vi "Tosca-Initialize Digital Inputs.vi"(7 "Action":enum16{"Stop", "Preview", "Run"}(ring), 11 "error in (no error)":errorcluster) -> (4 "Digital Inputs out":T1[](array[typedef]), 15 "error out":errorcluster)   [LabVIEW 2020]
uses:
  Tosca-Digital Input.ctl
  Sub VIs/Tosca-Globals.vi
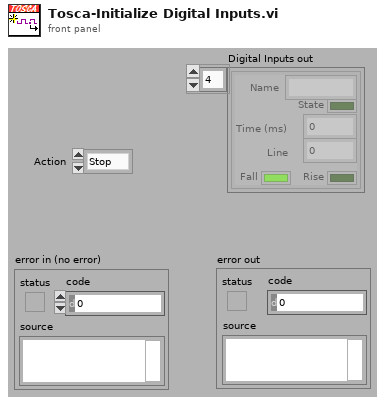
[diagram p1: front panel]
types:
  T1 = typedef "Tosca-Digital Input.ctl" = cluster{"Name":string, "State":bool, "Time (ms)":dbl, "Line":i32, "Rise":bool, "Fall":bool}
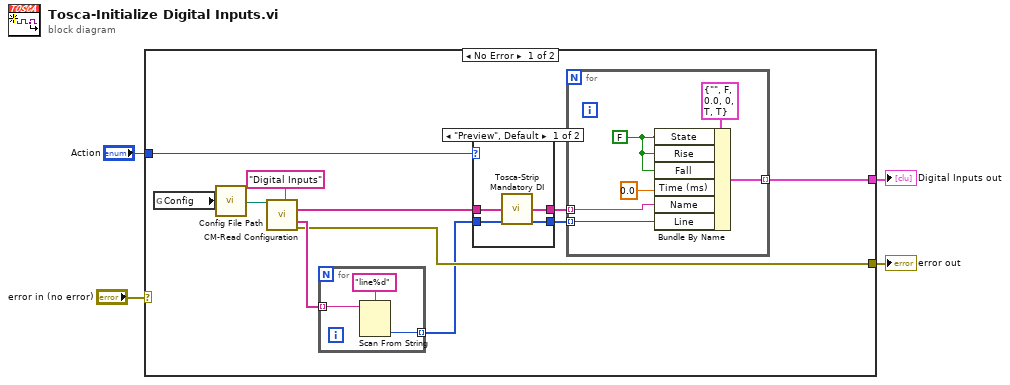
[diagram p0: block diagram]
diagram:
  n1 = case shown="No Error" "error in (no error)" {
    selector: "error in (no error)" -> [_ w31]
    tunnel: [w6 w31] -> w3
    tunnel: [w15 _] -> w2
    tunnel: "Action" -> [w14 _]
    frame No Error {
      n2 = global read "Tosca-Globals.vi" "Config"() -> (w11:string)
      n3 = call "Config File Path.vi"("AppName"=w11) -> ("Default config file name"=w9:path)
      n4 = call "CM-Read Configuration.vi"("Connection File Path"=w9, "Section"="Digital Inputs") -> ("Names"=w8:string[], "Devices"=w7:string[], "error out"=w6:errorcluster)  [unwired: 9 in, 2 out]
      n5 = for {
        tunnel: w7 -> [w18] mode=indexing
        tunnel: [w16] -> w5 mode=indexing
        n6 = Scan From String(format string="line%d", input string=w18) -> (output 1=w16:i32)  [unwired: 3 in, 3 out]
      }
      n7 = case shown="\"Preview\", Default" w14 {
        tunnel: [w20 w24] -> w13
        tunnel: w8 -> [w22 w24]
        tunnel: [w19 w23] -> w12
        tunnel: w5 -> [w21 w23]
        frame "Preview", Default {
          n8 = call "Tosca-Strip Mandatory DI.vi"("Digital Signals"=w22, "Lines"=w21) -> ("Filtered DI"=w20:string[], "Filtered Lines"=w19:i32[])  [unwired: 11 in, 1 out]
        }
        frame "Run" {
        }
      }
      n9 = for {
        tunnel: [w29] -> w15 mode=indexing
        tunnel: w13 -> [w26] mode=indexing
        tunnel: w12 -> [w25] mode=indexing
        w27 = FALSE ("State")
        n10 = Bundle By Name(cluster=T1 {"Name"="", "State"=FALSE, "Time (ms)"=0.0, "Line"=0, "Rise"=TRUE, "Fall"=TRUE} ("Digital Input"), "State"=w27, "Rise"=w27, "Fall"=w27, "Time (ms)"=0.0, "Name"=w26, "Line"=w25) -> (w29:T1)
      }
    }
    frame Error {
    }
  }
  "error out" <- w3
  "Digital Inputs out" <- w2
